vi "Example Barcode.vi"() -> ()   [LabVIEW 2020]
uses:
  g_ar_toolkit.image/g_ar_toolkit.image.lvlib
  g_ar_toolkit.feature_detection/BarcodeDetector/BarcodeDetector.lvclass
  g_ar_toolkit.image/ARGB Colour.ctl
  g_ar_toolkit.image/Font Face.ctl
  g_ar_toolkit.image/Text Drawing Settings.ctl
  g_ar_toolkit.image/ReadImageFileARGB.vi
  g_ar_toolkit.image/CreateEmptyImageARGB.vi
  g_ar_toolkit.image/DrawImageToPictureARGB.vi
  g_ar_toolkit.feature_detection/BarcodeDetector/DetectBarcodesARGB.vi
  g_ar_toolkit.image/DrawTextOnImageARGB.vi
  g_ar_toolkit.image/DrawPolyLinesOnImageARGB.vi
  g_ar_toolkit.common/Image Point (Integer).ctl
  g_ar_toolkit.common/g_ar_toolkit.common.lvlib
  g_ar_toolkit.feature_detection/BarcodeDetector/Detection Region.ctl
  g_ar_toolkit.feature_detection/BarcodeDetector/Detection.ctl
panel:
  out "Detections":T1[](array[typedef])
  out "Picture":picture
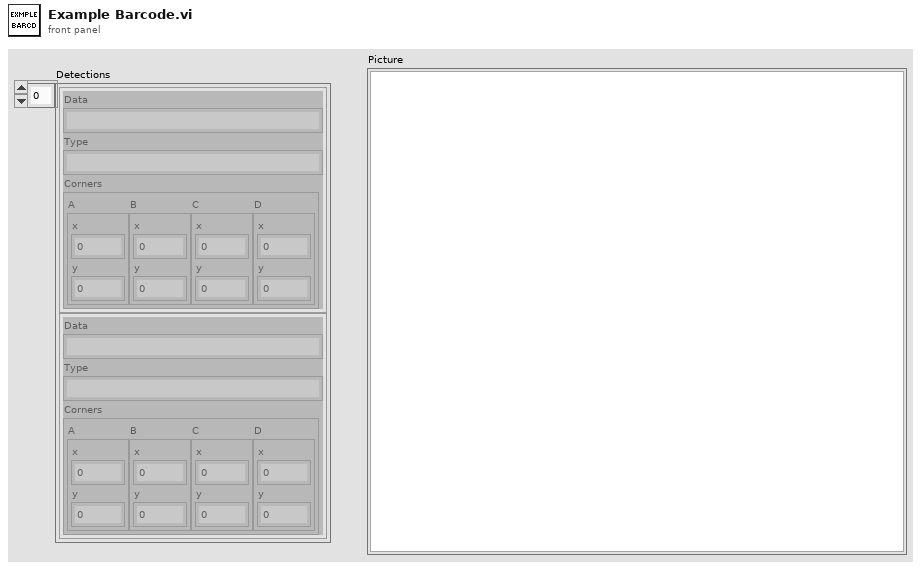
[diagram p1: front panel]
types:
  T1 = typedef "g_ar_toolkit.feature_detection.lvlib/BarcodeDetector.lvclass/Detection.ctl" = cluster{"Data":string, "Type":string, "Corners":T2}
  T2 = typedef "g_ar_toolkit.feature_detection.lvlib/BarcodeDetector.lvclass/Detection Region.ctl" = cluster{"A":T3, "B":T3, "C":T3, "D":T3}
  T3 = typedef "g_ar_toolkit.common.lvlib/Image Point (Integer).ctl" = cluster{"x":i32, "y":i32}
  T4 = typedef "g_ar_toolkit.image.lvlib/Text Drawing Settings.ctl" = cluster{"OpenCV Font Face":T5, "Font Scale":dbl}
  T5 = typedef "g_ar_toolkit.image.lvlib/Font Face.ctl" = enum8{"FONT_HERSHEY_SIMPLEX", "FONT_HERSHEY_PLAIN", "FONT_HERSHEY_DUPLEX", "FONT_HERSHEY_COMPLEX", "FONT_HERSHEY_TRIPLEX", "FONT_HERSHEY_COMPLEX_SMALL", "FONT_HERSHEY_SCRIPT_SIMPLEX", "FONT_HERSHEY_SCRIPT_COMPLEX", "FONT_ITALIC"}
  T6 = typedef "g_ar_toolkit.image.lvlib/ARGB Colour.ctl" = cluster{"Alpha":u8, "RGB":u32}
  T7 = typedef "g_ar_toolkit.feature_detection.lvlib/BarcodeDetector.lvclass/Detection Region Corners.ctl" = cluster{"A":T3, "B":T3, "C":T3, "D":T3}
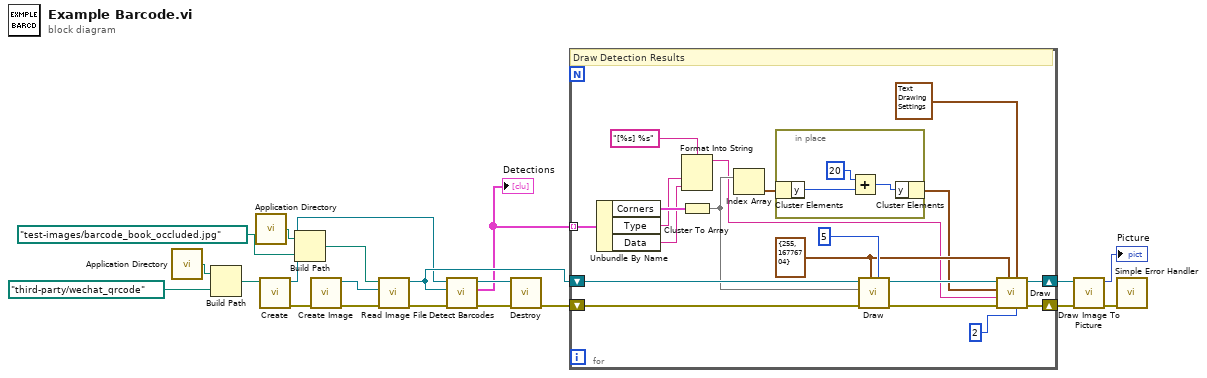
[diagram p0: block diagram]
diagram:
  n1 = call <vilib>:"Application Directory.vi"() -> ("Application Directory"=w15:path)
  n2 = Build Path(base path=w15, name or relative path=path "third-party/wechat_qrcode" ("Filepath")) -> (appended path=w3:path)
  n3 = call <vilib>:"Application Directory.vi"() -> ("Application Directory"=w18:path)
  n4 = call "Create.vi"("Super Resolution Model Directory (Default: Not A Path)"=w3) -> ("error out"=w1:errorcluster, "New BarcodeDetector"=w2:refnum<class "BarcodeDetector.lvclass">)  [unwired: 9 in]
  n5 = Build Path(base path=w18, name or relative path=path "test-images/barcode_book_occluded.jpg" ("Path")) -> (appended path=w17:path)
  n6 = call-poly "Create Image.vi"("error in (no error)"=w1) -> ("error out"=w14:errorcluster, "New ARGB Image"=w20:refnum<data-value>)  [unwired: 9 in]
  n7 = call-poly "Read Image File.vi"("error in (no error)"=w14, "ARGB Image Destination"=w20, "Filepath"=w17) -> ("error out"=w4:errorcluster, "ARGB Image Destination (duplicate)"=w11:refnum<data-value>)  [unwired: 7 in]
  n8 = call-poly "Detect Barcodes.vi"("error in (no error)"=w4, "ARGB Image"=w11, "BarcodeDetector in"=w2) -> ("error out"=w12:errorcluster, "Detections"=w10:T1[], "BarcodeDetector (Duplicate)"=w13:refnum<class "BarcodeDetector.lvclass">)  [unwired: 6 in]
  "Detections" <- w10
  n9 = call "Destroy.vi"("error in (no error)"=w12, "BarcodeDetector in"=w13) -> ("error out"=w9:errorcluster)  [unwired: 9 in]
  n10 = for {
    shift-right: [w31] -> w7
    shift-left: w11 -> [w39]
    tunnel: w10 -> [w38] mode=indexing
    shift-right: [w33] -> w8
    shift-left: w9 -> [w36]
    w30 = T6 {"Alpha"=255, "RGB"=16776704} ("ARGB Colour")
    # "Draw Detection Results"
    n11 = Unbundle By Name(w38) -> ("Corners"=w37:T7, "Type"=w28:string, "Data"=w29:string)
    n12 = Format Into String(format string="[%s] %s", w28, w29) -> (resulting string=w25:string)  [unwired: 2 in, 1 out]
    n13 = Cluster To Array(cluster=w37) -> (array=w26:T3[])
    n14 = Index Array(array=w26) -> (element=w23:T3)  [unwired: 1 in]
    n15 = in-place {
      n16 = in-place-cluster #1(w23) -> ("y"=w42:i32)
      n17 = Add(x=20, y=w42) -> (x+y=w41:i32)
      n18 = in-place-cluster #1("y"=w41) -> (w22:T3)
    }
    n19 = call-poly "Draw.vi"("Thickness (Default: 1)"=5, "ARGB Colour"=w30, "error in (no error)"=w36, "Points"=w26, "ARGB Image"=w39) -> ("error out"=w35:errorcluster, "ARGB Image (Duplicate)"=w32:refnum<data-value>)  [unwired: 5 in]
    n20 = call-poly "Draw.vi"("Thickness (Default: 1)"=2, "Text Drawing Settings (Default: Simplex)"=T4 {"OpenCV Font Face"=enum."FONT_HERSHEY_SIMPLEX", "Font Scale"=0.6}, "ARGB Colour"=w30, "error in (no error)"=w35, "Text"=w25, "Origin"=w22, "ARGB Image"=w32) -> ("error out"=w33:errorcluster, "ARGB Image (Duplicate)"=w31:refnum<data-value>)  [unwired: 3 in]
  }
  n21 = call-poly "Draw Image To Picture.vi"("error in (no error)"=w8, "ARGB Image Source"=w7) -> ("error out"=w6:errorcluster, "Picture"=→"Picture":picture)  [unwired: 8 in]
  n22 = call <vilib>:"Simple Error Handler.vi"("error in (no error)"=w6) -> ()  [unwired: 4 in, 5 out]
